vi "Get or Create App Directory.vi"(8 "error in (no error)":errorcluster, 11 "Relative Path":path) -> (0 "error out":errorcluster, 3 "Ouput File Path":path)   [LabVIEW 2020, in "RxnRover.lvlib" / "File IO.lvlib" / "Project Locations.lvlib"]
doc: "Create or access a local app directory given a relative path(String) EX: appname/appdirectory\n\nLocates the correct system-specfic base directory for state data %LOCALAPPDATA(WIndows) or $XDG_STATE_HOME(Linux) or ~/Library/Application Support(Mac OS) and appends the relative path\nCreates the directory if it does not exist. \nCompliant with XKG Base Directory Specification \n\nCreated 5/20/2025 - Labview 2020\nRxnRover"
uses:
  Project Locations/Project Locations.lvlib
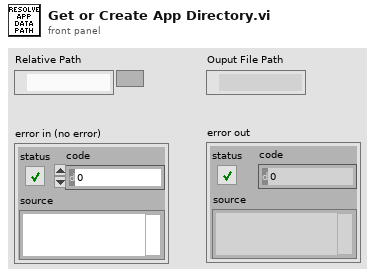
[diagram p1: front panel]
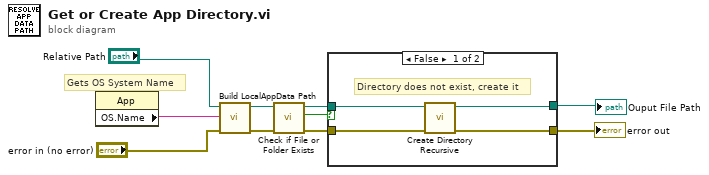
[diagram p0: block diagram]
diagram:
  # "Gets OS System Name"
  n1 = property class="App"() -> ("OS.Name"=w2:string)  [unwired: 2 in, 2 out]
  n2 = call "Build LocalAppData Path.vi"("error in (no error)"="error in (no error)", "Operating System"=w2, "Relative path"="Relative Path") -> ("error out"=w6:errorcluster, "Full Path"=w10:path)  [unwired: 7 in]
  n3 = call <vilib>:"Check if File or Folder Exists.vi"("error in (no error)"=w6, "path"=w10) -> ("error out"=w7:errorcluster, "file or folder exists?"=w9:bool, "dup path"=w8:path)  [unwired: 7 in]
  n4 = case shown="False" w9 {
    tunnel: w8 -> [w14 w16]
    tunnel: [w13 w16] -> w3
    tunnel: w7 -> [w12 w15]
    tunnel: [w11 w15] -> w4
    frame False {
      # "Directory does not exist, create it"
      n5 = call <vilib>:"Create Directory Recursive.vi"("error in (no error)"=w12, "directory"=w14) -> ("error out"=w11:errorcluster, "directory copy"=w13:path)  [unwired: 3 in, 1 out]
    }
    frame True {
      # "Directory already exists pass the full path"
    }
  }
  "error out" <- w4
  "Ouput File Path" <- w3
